vi "Approach_percentDecrease_VUW.vi"(7 "Computer called (T/F)":bool) -> ()   [LabVIEW 2023]
uses:
  Sub_Vi/TypeDefsControls/Zposition.ctl
  Sub_Vi/TypeDefsControls/Piezo Velocity.ctl
  Sub_Vi/TypeDefsControls/Voltage.ctl
  Sub_Vi/TypeDefsControls/Xposition.ctl
  Sub_Vi/TypeDefsControls/Yposition.ctl
  Sub_Vi/TypeDefs/WayPointCluster.ctl
  Sub_Vi/TypeDefs/ChangeOnFly.ctl
  Sub_Vi/TypeDefs/Settings.ctl
  Sub_Vi/TypeDefs/Display.ctl
  Sub_Vi/TypeDefsControls/Feedback Type.ctl
  Settings.vi
panel:
  out "Precent Change for feedback (percent) 2":dbl=2.0
  out "Current 1":cluster{"Y":dbl[], "Y":dbl[]}[](graph)
  in  "Boolean Negative":bool
  in  "Boolean Positive":bool=TRUE
  in  "Feedback Type":T1=enum."Current 1"
  in  "Display Cluster":T2
  in  "SettingsCluster":T3={"Sample Rate (us)"=1, "Samples Per Data Point (int, power of 2)"=1000, "DistanceToBulk (um)"=-1.0, "HoldTimeScaler"=1, "SaveData"=TRUE, "DistanceToBulk (um) 2"=-1.0, "DistanceToBulk (um) 3"=-1.0}
  in  "ChangeonFly":T4
  in  "WayPointCluster":T5
  in  "Start scan Button":bool
  in  "Stop":bool
  in  "Pause":bool
  in  "Threshold (percent)":dbl=2.0
  in  "Set X":bool
  in  "Set Y":bool
  in  "Y":T6=100.0 min=0.0 max=100000.0
  in  "X":T7=100.0 min=0.0 max=100000.0
  in  "Approach Voltage (V)":T8 min=-10.0 max=10.0
  in  "Approach Rate (µm/s)":T9=0.1 min=0.0
  in  "End Extension (µm)":T10 min=0.0 max=100000.0
  in  "Start Extention (µm)":T10=150.0 min=0.0 max=100000.0
  out "?":cluster{"Y":dbl[], "Y":dbl[]}[](graph)
  out "?":dbl[](graph)
  # "Settings"
  # "Pause at"
  # "Advanced Settings"
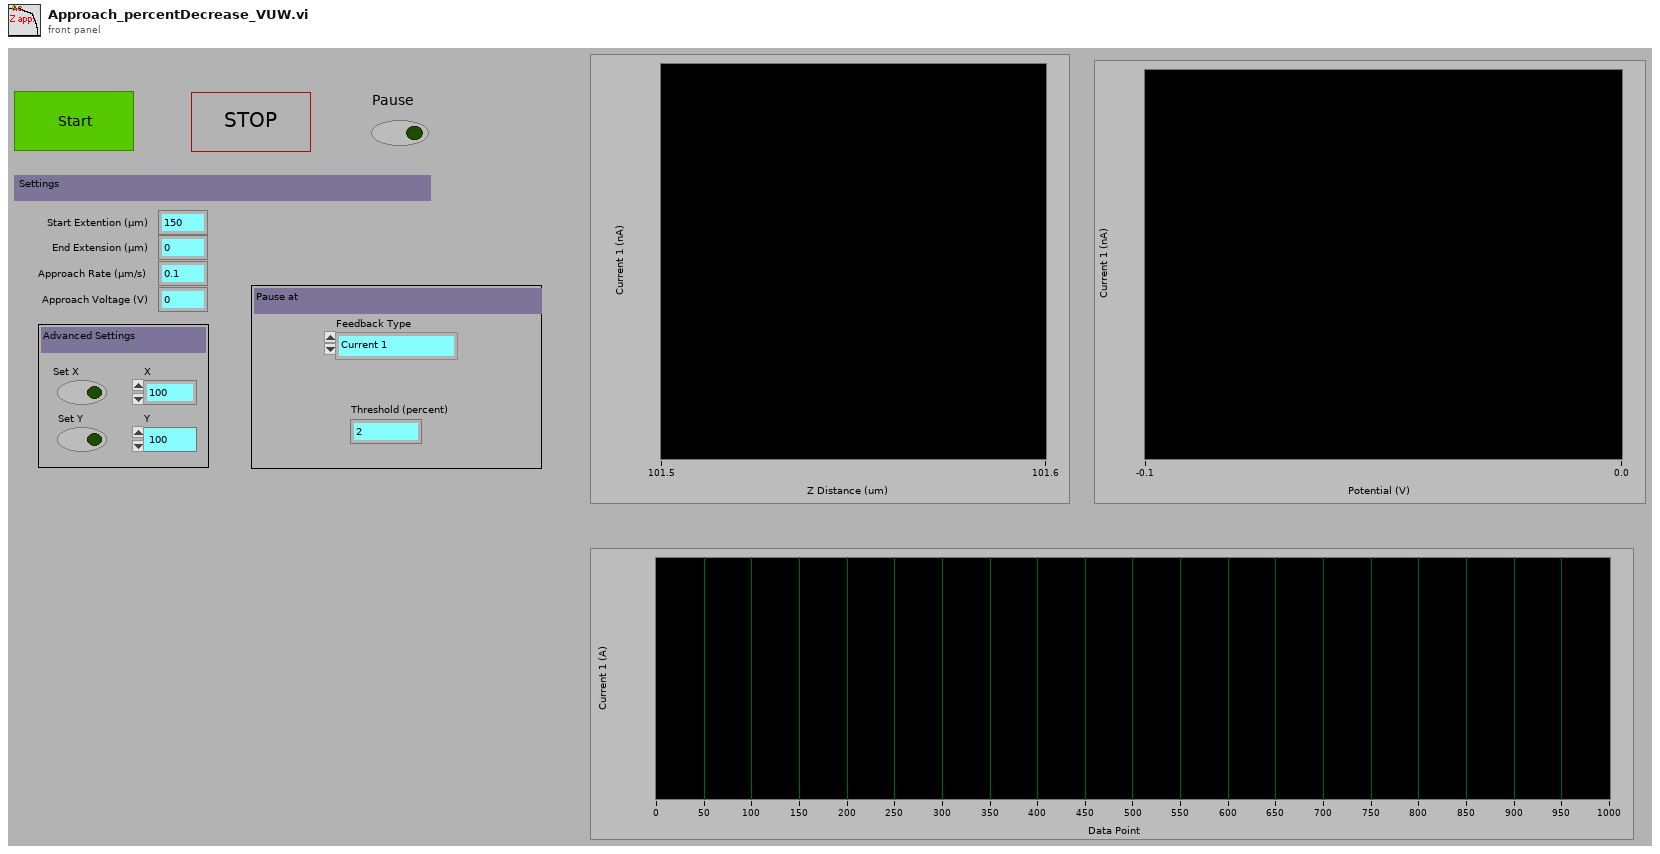
[diagram p1: front panel]
types:
  T1 = typedef "Feedback Type.ctl" = enum16{"AC Magnitude", "Current 1", "Current 2", "Phase"}
  T2 = typedef "Display.ctl" = cluster{"X":refnum<vi>, "Y":refnum<vi>, "Z":refnum<vi>, "Amp":refnum<vi>, "Phase":refnum<vi>, "t vs Z":refnum<vi>, "t vs C1":refnum<vi>, "t vs C2":refnum<vi>, "t vs C3":refnum<vi>, "t vs Amp":refnum<vi>, "t vs Phase":refnum<vi>, "t vs X":refnum<vi>, "t vs Y":refnum<vi>, "Z vs C1":refnum<vi>, "Z vs C2":refnum<vi>, "Z vs C3":refnum<vi>, "V vs C1":refnum<vi>, "V vs C2":refnum<vi>, "V vs C3":refnum<vi>, "X/Y/Z F":refnum<vi>, "X/Y/Z R":refnum<vi>, "X/Y/C1 F":refnum<vi>, "X/Y/C1 R":refnum<vi>, "X/Y/C2 F":refnum<vi>, "X/Y/C2 R":refnum<vi>, "X/Y/C3 F":refnum<vi>, "X/Y/C3 R":refnum<vi>, "NumberOfLines":u16, "um Per Pixel":dbl, "um Per Line":dbl, "X Center":dbl, "Hop X/Y/Z":refnum<vi>, "Hop X/Y/C1":refnum<vi>, "Hop X/Y/C2":refnum<vi>, "Hop X/Y/C3":refnum<vi>, "X Width":dbl, "Y Width":dbl, "Hopping Distance":dbl, "V2 vs C1":refnum<vi>, "V vs Phase":refnum<vi>, "Y Center":dbl, "Number of Pixels":dbl, "V2 vs C2":refnum<vi>, "V2 vs C3":refnum<vi>, "V vs y":refnum<vi>, "V2 vs y":refnum<vi>, "Z vs Amp":refnum<vi>, "Z vs Phase":refnum<vi>}
  T3 = typedef "Settings.ctl" = cluster{"Sample Rate (us)":u32, "Samples Per Data Point (int, power of 2)":i16, "DistanceToBulk (um)":dbl, "HoldTimeScaler":u64, "SaveData":bool, "DistanceToBulk (um) 2":dbl, "DistanceToBulk (um) 3":dbl}
  T4 = typedef "ChangeOnFly.ctl" = cluster{"Stop (boolean)":refnum<vi>, "Pause (boolean)":refnum<vi>, "EndCurrentLine (boolean)":refnum<vi>, "max movement per update step (Interger, nm)":refnum<vi>, "P (float, arb)":refnum<vi>, "Feedback set point (double, Amps)":refnum<vi>, "Voltage (double, V)":refnum<vi>, "Feedback set point 2 (double, Amps)":refnum<vi>, "Stop on Greater Than 2? (boolean)":refnum<vi>, "Stop on Greater Than? (boolean)":refnum<vi>, "Voltage 2 (double, V)":refnum<vi>, "Feedback Type (enum)":refnum<vi>, "Feedback Type 2 (enum)":refnum<vi>}
  T5 = typedef "WayPointCluster.ctl" = cluster{"X (um)":dbl[], "Y (um)":dbl[], "Z (um)":dbl[], "V (V)":dbl[], "X Velocity (um s-1)":dbl[], "Y Velocity (um s-1)":dbl[], "Z Velocity (um s-1)":dbl[], "V Velocity (V s-1)":dbl[], "FeedBack Type (enum)":u16[], "Move X (boolean)":bool[], "Move Y (boolean)":bool[], "Move Z (boolean)":bool[], "Move V (boolean)":bool[], "Jump V (boolean)":bool[], "Hold (boolean)":bool[], "Hold Time":u32[], "V2 (V)":dbl[], "Move V2":bool[], "V2 Velocity (V s-1)":dbl[], "Jump V2 (boolean)":bool[], "Update z Position delta (ms)":i16[], "Hold Feedback1":bool[], "Move Z PicoMotor":bool[], " Z PicoMotor Direction":bool[], "DIO0":bool[]}
  T6 = typedef "Yposition.ctl" = dbl
  T7 = typedef "Xposition.ctl" = dbl
  T8 = typedef "Voltage.ctl" = dbl
  T9 = typedef "Piezo Velocity.ctl" = dbl
  T10 = typedef "Zposition.ctl" = dbl
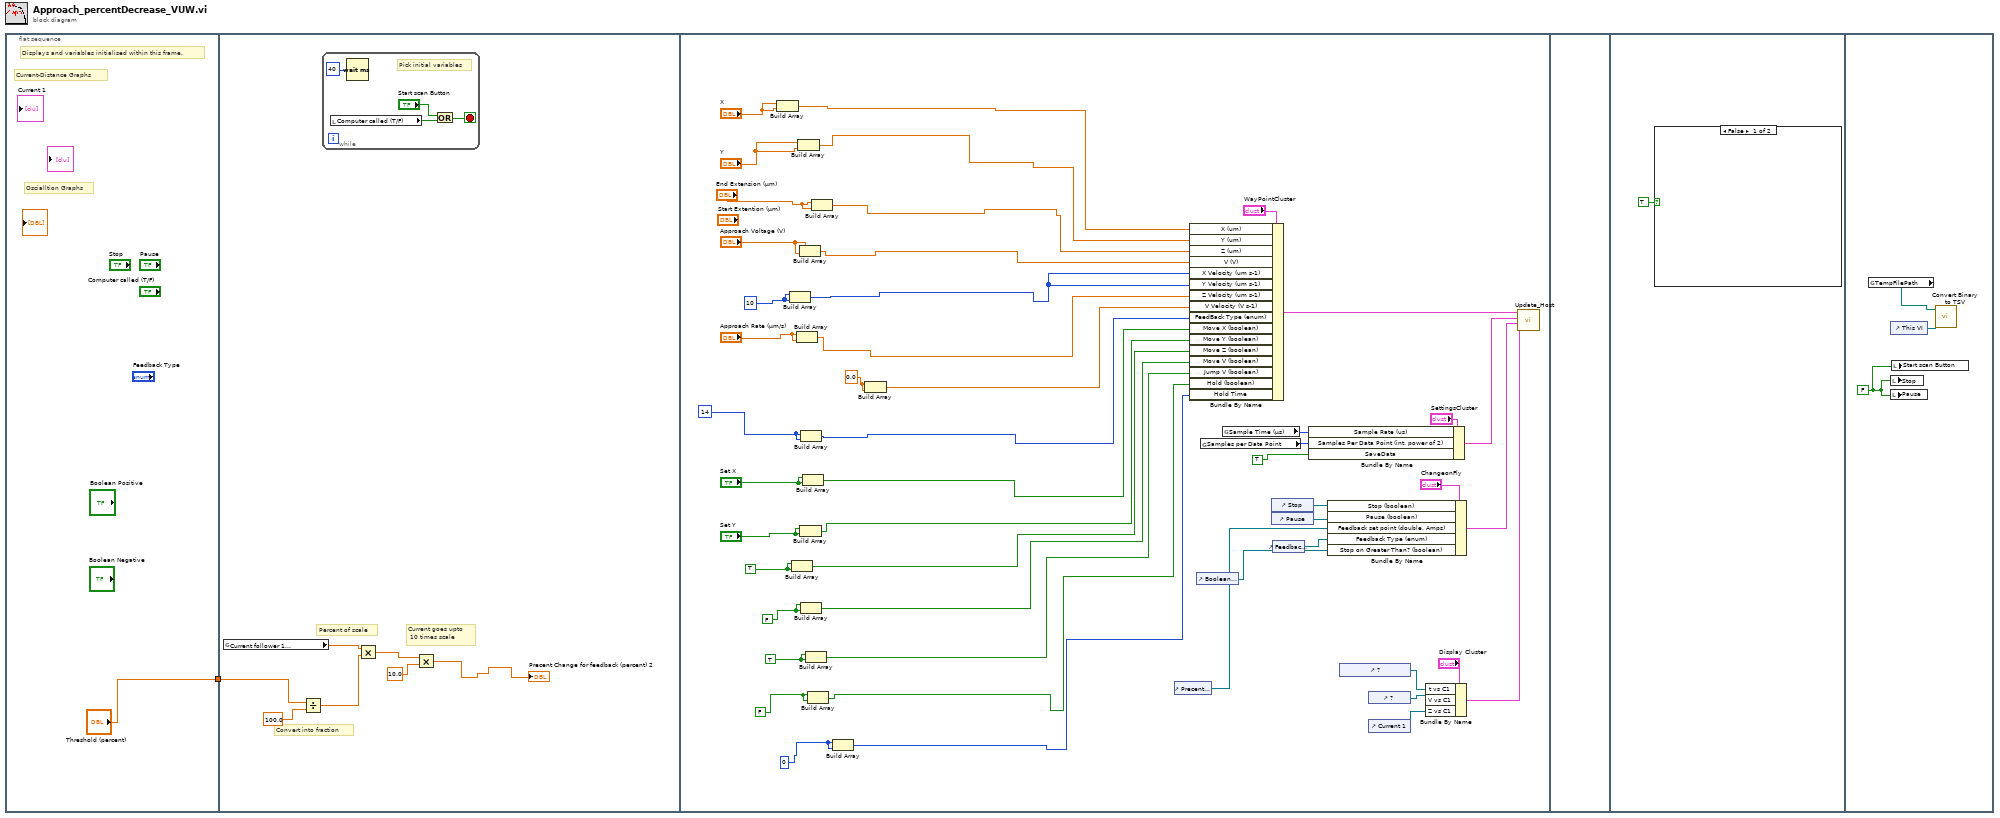
[diagram p0: block diagram]
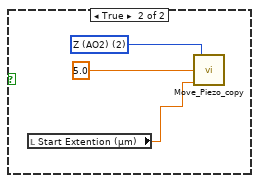
[diagram p2: hidden frame]
diagram:
  n1 = flat-sequence {
    tunnel: ["Threshold (percent)"] -> w1
    tunnel: w1 -> [w4]
    frame #0 {
      # "Oscialltion Graphs"
      # "Current-Distance Graphs"
      # "Displays and variables initialised within this frame."
    }
    frame #1 {
      # "Current goes upto\n 10 times scale"
      # "Percent of scale"
      # "Convert into fraction"
      n2 = global read "Settings.vi" "Current follower 1\n (AI-3)"() -> (w7:dbl)
      n3 = Divide(x=w4, y=100.0) -> (x/y=w6:dbl)
      n4 = while {
        stop <- w13 stop-if-true
        # "Pick initial variables"
        n5 = local read "Computer called (T/F)"() -> (w11:bool)
        n6 = Wait (ms)(milliseconds to wait=u32 40) -> ()  [unwired: 1 out]
        n7 = Or(x="Start scan Button", y=w11) -> (x .or. y?=w13:bool)
      }
      n8 = Multiply(x=w7, y=w6) -> (x*y=w8:dbl)
      n9 = Multiply(x=w8, y=10.0) -> (x*y=→"Precent Change for feedback (percent) 2":dbl)
    }
    frame #2 {
      w21 = u16 14 ("Approach Type")
      w14 = u32 0 ("element")
      w16 = TRUE ("Set Z")
      w17 = FALSE ("element")
      w22 = 0.0
      w15 = FALSE ("Set Z")
      w18 = TRUE ("Set Z")
      w24 = 10
      n10 = Build Array("X", "X") -> (w44:T7[])
      n11 = Build Array(w24, w24) -> (w40:i32[])
      n12 = Build Array(w18, w18) -> (w34:bool[])
      n13 = Build Array("Approach Rate (µm/s)", "Approach Rate (µm/s)") -> (w39:T9[])
      n14 = Build Array("Y", "Y") -> (w43:T6[])
      n15 = Build Array("Approach Voltage (V)", "Approach Voltage (V)") -> (w41:T8[])
      n16 = Build Array("Set Y", "Set Y") -> (w35:bool[])
      n17 = Build Array(w21, w21) -> (w37:u16[])
      n18 = Build Array(w17, w17) -> (w33:bool[])
      n19 = Build Array("Set X", "Set X") -> (w36:bool[])
      n20 = Build Array(w16, w16) -> (w32:bool[])
      n21 = Build Array(w15, w15) -> (w31:bool[])
      n22 = Build Array("End Extension (µm)", "End Extension (µm)") -> (w42:T10[])
      n23 = Build Array(w14, w14) -> (w30:u32[])
      n24 = Build Array(w22, w22) -> (w38:dbl[])
      n25 = control-ref of="Precent Change for feedback (percent) 2"() -> (w29:refnum<vi>)
      n26 = Bundle By Name(cluster="WayPointCluster", "X (um)"=w44, "Y (um)"=w43, "Z (um)"=w42, "V (V)"=w41, "X Velocity (um s-1)"=w40, "Y Velocity (um s-1)"=w40, "Z Velocity (um s-1)"=w39, "V Velocity (V s-1)"=w38, "FeedBack Type (enum)"=w37, "Move X (boolean)"=w36, "Move Y (boolean)"=w35, "Move Z (boolean)"=w34, "Move V (boolean)"=w33, "Jump V (boolean)"=w32, "Hold (boolean)"=w31, "Hold Time"=w30) -> (w62:T5)
      n27 = control-ref of="Boolean Positive"() -> (w46:refnum<vi>)
      n28 = global read "Settings.vi" "Samples per Data Point"() -> (w53:u16)
      n29 = global read "Settings.vi" "Sample Time (µs)"() -> (w54:u32)
      n30 = control-ref of="Stop"() -> (w58:refnum<vi>)
      n31 = control-ref of="Pause"() -> (w57:refnum<vi>)
      n32 = control-ref of="Feedback Type"() -> (w47:refnum<vi>)
      n33 = Bundle By Name(cluster="SettingsCluster", "Sample Rate (us)"=w54, "Samples Per Data Point (int, power of 2)"=w53, "SaveData"=TRUE) -> (w60:T3)
      n34 = Bundle By Name(cluster="ChangeonFly", "Stop (boolean)"=w58, "Pause (boolean)"=w57, "Feedback set point (double, Amps)"=w29, "Feedback Type (enum)"=w47, "Stop on Greater Than? (boolean)"=w46) -> (w59:T4)
      n35 = control-ref of="?"() -> (w45:refnum<vi>)
      n36 = control-ref of="?"() -> (w52:refnum<vi>)
      n37 = control-ref of="Current 1"() -> (w51:refnum<vi>)
      n38 = Bundle By Name(cluster="Display Cluster", "t vs C1"=w45, "V vs C1"=w52, "Z vs C1"=w51) -> (w61:T2)
      n39 = call "Update_Host.vi"("Display Cluster"=w61, "ChangeonFly"=w59, "SettingsCluster"=w60, "WayPointCluster"=w62) -> ()  [unwired: 6 in]
    }
    frame #3 {
    }
    frame #4 {
      n40 = case shown="False" TRUE {
        frame False {
        }
        frame True {
          w66 = u16 2 items=["X (AO0)", "Y (AO1)", "Z (AO2)", "V (AO3)", "V2 (AO4)"] ("Piezo")
          n41 = local read "Start Extention (µm)"() -> (w64:T10)
          n42 = call "Move_Piezo_copy.vi"("Piezo"=w66, "Movement Speed (µm/s)"=5.0 ("Scan Rate (um/s)"), "Position (µm) (or V)"=w64) -> ()  [unwired: 13 in]
        }
      }
    }
    frame #5 {
      w68 = FALSE ("Start Scanning Button")
      n43 = global read "Settings.vi" "TempFilePath"() -> (w67:path)
      n44 = control-ref of="This VI"() -> (w69:refnum<vi>)
      n45 = local write "Stop"(w68) -> ()
      n46 = local write "Pause"(w68) -> ()
      n47 = local write "Start scan Button"(w68) -> ()
      n48 = call "Convert Binary to TSV.vi"("This VI"=w69, "TDMS DataFile Name"=w67) -> ()  [unwired: 10 in]
    }
  }
